vi "Voltage2Temperature.vi"(8 "Referencni telpota":dbl, 9 "Typ termoclanku":u16(ring) items=["J", "K", "T"], 10 "Vstupni napeti":dbl) -> (3 "Vystupni teplota":dbl)   [LabVIEW 2022 SP3]
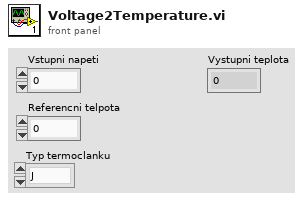
[diagram p1: front panel]
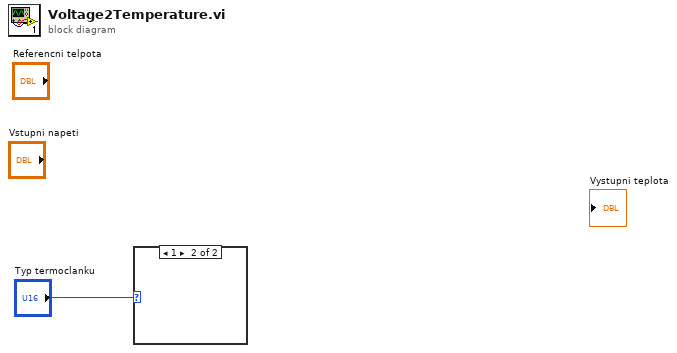
[diagram p0: block diagram]
diagram:
  n1 = case shown="1" "Typ termoclanku" {
    frame 0, Default {
    }
    frame 1 {
    }
  }
